vi "Periodictable.vi"(0 "Path":path) -> (7 "S1":dbl[](array[numeric]), 10 "Periodic":string[][](array[string]), 12 "Element":string[](array[string]), 13 "Array 3":dbl[](array[numeric]), 14 "S4":dbl[](array[numeric]), 15 "Array 6":dbl[](array[numeric]), 16 "S3":dbl[](array[numeric]), 17 "Array 5":dbl[](array[numeric]), 18 "S2":dbl[](array[numeric]), 19 "Array 4":dbl[](array[numeric]))   [LabVIEW 2012]
uses:
  <vilib>/Utility/file.llb/Read From Spreadsheet File (string).vi
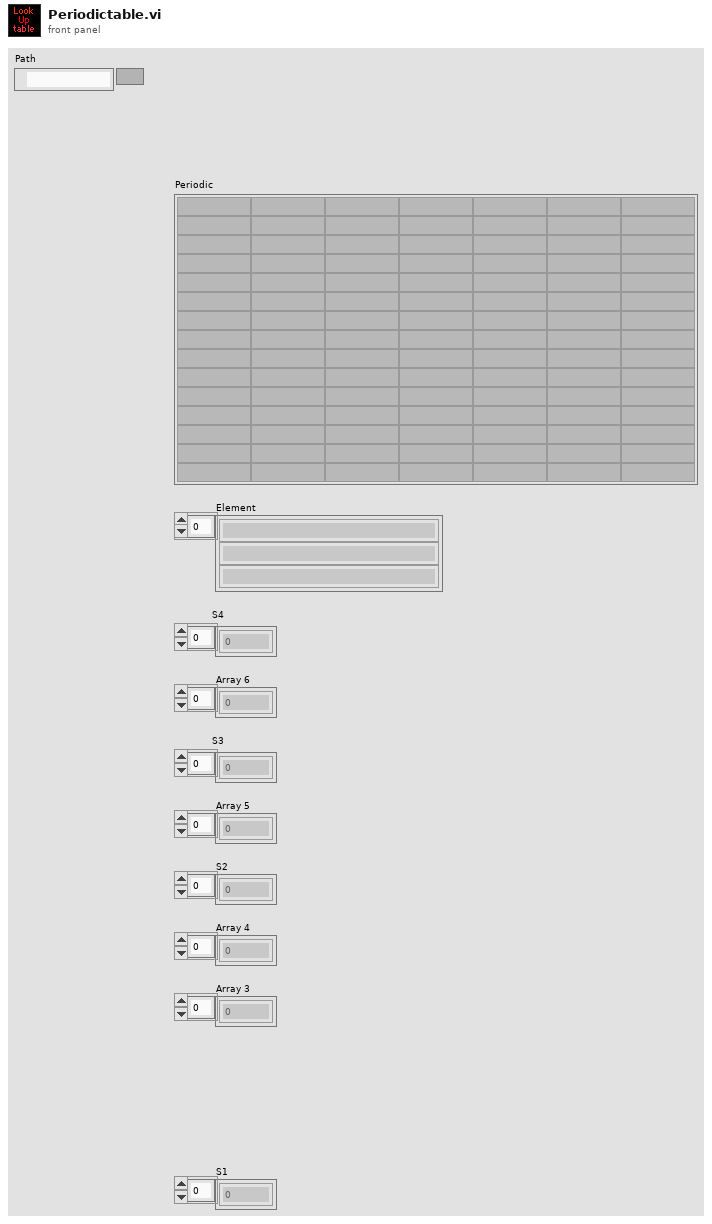
[diagram p1: front panel]
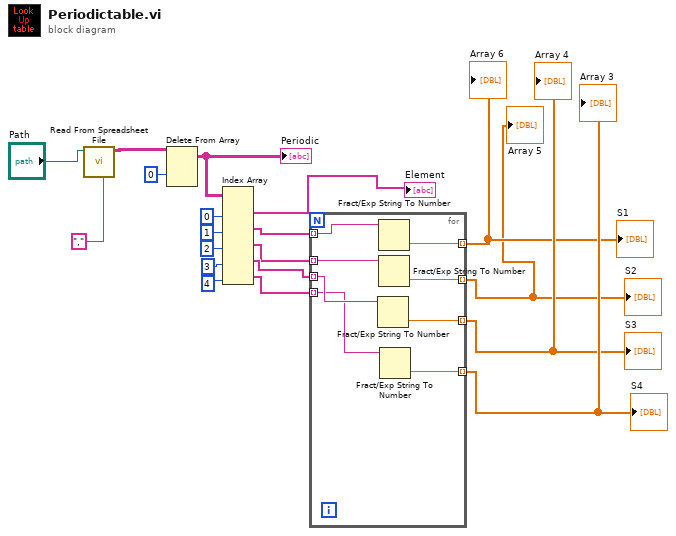
[diagram p0: block diagram]
diagram:
  n1 = call-poly <vilib>:"Read From Spreadsheet File.vi"("delimiter (\\t)"="," ("delimiter (\\t)"), "file path (dialog if empty)"="Path") -> ("all rows"=w2:string[][])  [unwired: 5 in, 4 out]
  n2 = Delete From Array(array=w2, index (row)=0) -> (array with subset deleted=w18:string[][])  [unwired: 2 in, 1 out]
  "Periodic" <- w18
  n3 = Index Array(array=w18, index (col) #1=0 ("disabled index (col)"), index (col) #2=1 ("index (col)"), index (col) #3=2 ("index (col)"), index (col) #4=3 ("index (col)"), index (col) #5=4 ("index (col)")) -> (element #1=→"Element":string[], element #2=w9:string[], element #3=w10:string[], element #4=w13:string[], element #5=w14:string[])  [unwired: 5 in]
  n4 = for {
    tunnel: w9 -> [w27] mode=indexing
    tunnel: w10 -> [w26] mode=indexing
    tunnel: [w25] -> w15 mode=indexing
    tunnel: [w24] -> w1 mode=indexing
    tunnel: [w23] -> w16 mode=indexing
    tunnel: w13 -> [w22] mode=indexing
    tunnel: w14 -> [w21] mode=indexing
    tunnel: [w20] -> w17 mode=indexing
    n5 = Fract/Exp String To Number(string=w22) -> (number=w23:dbl)  [unwired: 3 in, 1 out]
    n6 = Fract/Exp String To Number(string=w27) -> (number=w25:dbl)  [unwired: 3 in, 1 out]
    n7 = Fract/Exp String To Number(string=w26) -> (number=w24:dbl)  [unwired: 3 in, 1 out]
    n8 = Fract/Exp String To Number(string=w21) -> (number=w20:dbl)  [unwired: 3 in, 1 out]
  }
  "S1" <- w15
  "S2" <- w1
  "S3" <- w16
  "S4" <- w17
  "Array 3" <- w17
  "Array 4" <- w16
  "Array 5" <- w1
  "Array 6" <- w15
